vi "position sweep(SubVI).vi"(0 "data":refnum<queue>, 2 "Instrument Ref In":refnum<k24>, 4 "config":refnum<queue>, 5 "steps number":i32, 7 "ch str":string, 9 "Position":dbl=300.0, 12 "Resource In":refnum<visa-resource-name>, 13 "Position 2":dbl=300.0, 14 "Speed":i32=10 min=0 max=14) -> (8 "错误输出":errorcluster)   [LabVIEW 2019, in "SubVI.lvlib"]
uses:
  SubVI.lvlib
  lib/QDInstrument.dll
  config.ctl
panel:
  # "(真是通道1，假是通道2)"
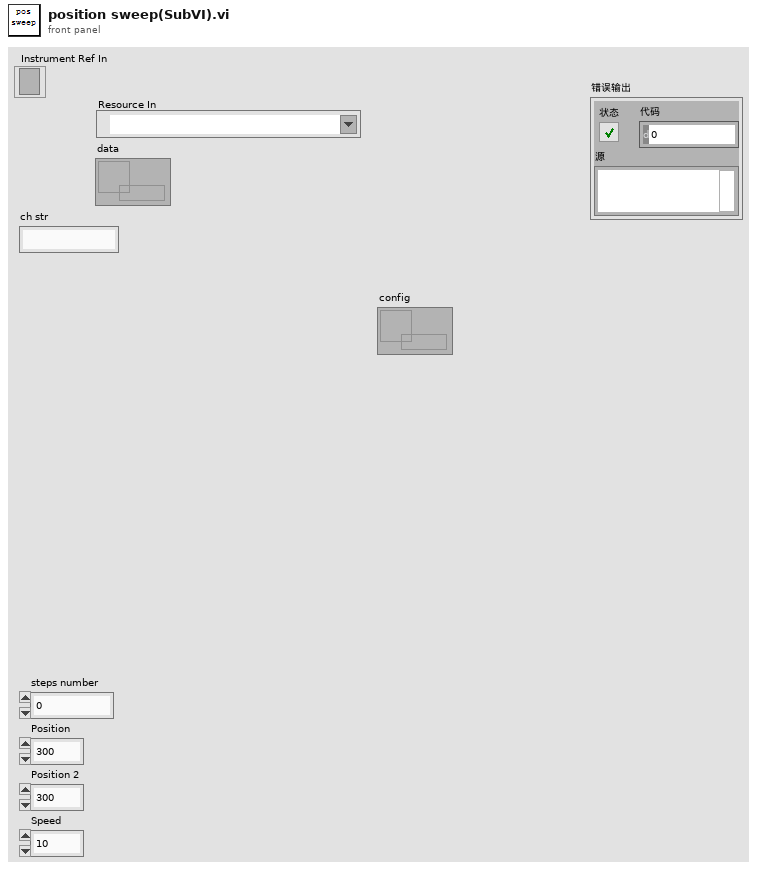
[diagram p1: front panel]
types:
  T1 = typedef "config.ctl" = cluster{"error":bool, "initialize":string, "数值":dbl, "6221":cluster{"6221 Resource":refnum<visa-resource-name>, "Delta status":bool}, "7001":cluster{"Ch":bool}}
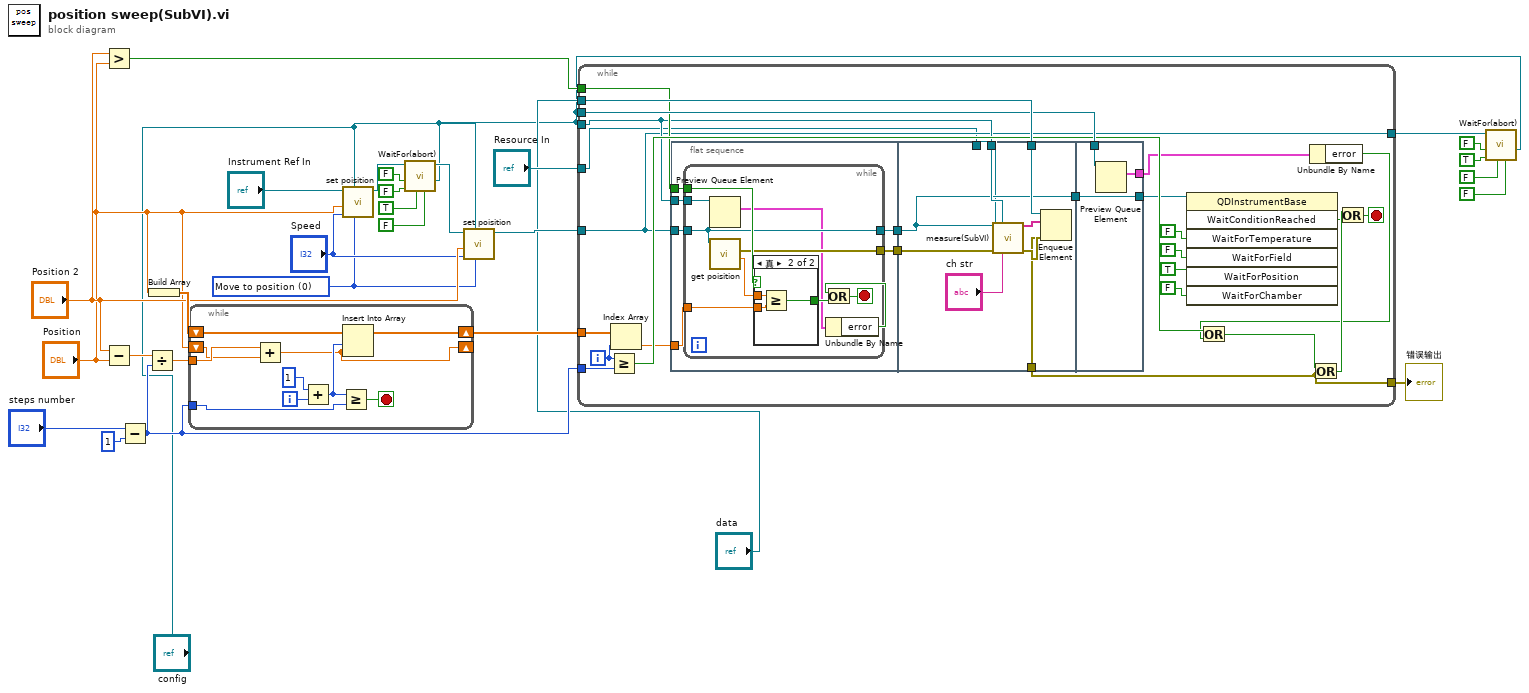
[diagram p0: block diagram]
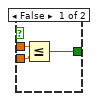
[diagram p2: hidden frame]
diagram:
  w4 = u16 0 items=["Move to position", "Move to limit", "Redefine current position"] ("Mode")
  n1 = Greater?(x="Position 2", y="Position") -> (0:w17:bool)
  n2 = Subtract(x="Position 2", y="Position") -> (x-y=w29:dbl)
  n3 = Subtract(x="steps number", y=1) -> (x-y=w6:i32)
  n4 = Divide(x=w29, y=w6) -> (x/y=w27:dbl)
  n5 = Build Array("Position") -> (w28:dbl[])
  n6 = while {
    shift-right: [w39] -> w19
    shift-left: w28 -> [w38]
    tunnel: w27 -> [w33]
    tunnel: w6 -> [w32]
    shift-right: [w31] -> _
    shift-left: "Position" -> [w30]
    i -> [w37]
    stop <- w34 stop-if-true
    n7 = Add(x=w33, y=w30) -> (x+y=w31:dbl)
    n8 = Add(x=1, y=w37) -> (x+y=w35:i32)
    n9 = Greater Or Equal?(x=w35, y=w32) -> (x >= y?=w34:bool)
    n10 = Insert Into Array(array=w38, index=w35, new element=w31) -> (w39:dbl[])
  }
  n11 = call "set poisition.vi"("Mode"=w4, "config"="config", "Slow down code\ndefault = 0"="Speed", "Position (deg)"="Position", "Instrument Ref In"="Instrument Ref In") -> ("Instrument Ref Out"=w5:refnum<k24>)  [unwired: 3 in, 1 out]
  n12 = call "WaitFor(abort).vi"("config"="config", "Wait For Chamber"=FALSE, "Wait For Position"=TRUE, "Wait For Field"=FALSE, "Wait For Temperature"=FALSE, "Instrument Ref In"=w5) -> ("Instrument Ref Out"=w20:refnum<k24>)  [unwired: 4 in, 1 out]
  n13 = call "set poisition.vi"("Mode"=w4, "config"="config", "Slow down code\ndefault = 0"="Speed", "Position (deg)"="Position 2", "Instrument Ref In"=w20) -> ("Instrument Ref Out"=w15:refnum<k24>)  [unwired: 3 in, 1 out]
  n14 = while {
    tunnel: w19 -> [w65]
    tunnel: w6 -> [w60]
    tunnel: "data" -> [w63]
    tunnel: "config" -> [w62]
    tunnel: w15 -> [w53]
    tunnel: w17 -> [w58]
    tunnel: [w53] -> w10
    tunnel: "config" -> [w56]
    tunnel: [w42] -> w9
    tunnel: "Resource In" -> [w43]
    i -> [w59]
    stop <- w47 stop-if-true
    n15 = Greater Or Equal?(x=w59, y=w60) -> (x >= y?=w61:bool)
    n16 = Index Array(array=w65, index=w59) -> (element=w57:dbl)
    n17 = flat-sequence {
      tunnel: [w68] -> w64
      tunnel: w53 -> [w71]
      tunnel: w58 -> [w70]
      tunnel: w57 -> [w69]
      tunnel: w56 -> [w67]
      tunnel: [w66] -> w55
      tunnel: w64 -> [w93]
      tunnel: w63 -> [w96]
      tunnel: w56 -> [w95]
      tunnel: [w89] -> w42
      tunnel: w55 -> [w91]
      tunnel: [w93] -> w51
      tunnel: w43 -> [w92]
      tunnel: w62 -> [w99]
      tunnel: [w98] -> w41
      tunnel: [w97] -> w52
      tunnel: w51 -> [w97]
      frame #0 {
        n18 = while {
          tunnel: w71 -> [w79]
          tunnel: w70 -> [w81]
          tunnel: w69 -> [w80]
          tunnel: [w79] -> w68
          tunnel: w67 -> [w77]
          tunnel: [w75] -> w66
          stop <- w72 stop-if-true
          n19 = Preview Queue Element(queue=w77) -> (element=w74:T1)  [unwired: 2 in, 3 out]
          n20 = call "get poisition.vi"("Instrument Ref In"=w79) -> ("Position"=w78:dbl, "error out"=w75:errorcluster)  [unwired: 4 in, 1 out]
          n21 = case shown="真" w81 {
            tunnel: w78 -> [w84 w87]
            tunnel: w80 -> [w83 w86]
            tunnel: [w82 w85] -> w76
            frame False {
              n22 = Less Or Equal?(x=w84, y=w83) -> (x <= y?=w82:bool)
            }
            frame True {
              n23 = Greater Or Equal?(x=w87, y=w86) -> (x >= y?=w85:bool)
            }
          }
          n24 = Unbundle By Name(w74) -> ("error"=w73:bool)
          n25 = Or(x=w73, y=w76) -> (x .or. y?=w72:bool)
        }
      }
      frame #1 {
        n26 = call "measure(SubVI).vi"(".NET引用句柄输入"=w93, "config"=w95, 7:w92, "error in (no error)"=w91, "ch str"="ch str") -> ("data"=w94:string[], "error out"=w90:errorcluster)  [unwired: 9 in]
        n27 = Enqueue Element(queue=w96, element=w94, error in (no error)=w90) -> (error out=w89:errorcluster)  [unwired: 1 in, 2 out]
      }
      frame #2 {
        n28 = Preview Queue Element(queue=w99) -> (element=w98:T1)  [unwired: 2 in, 3 out]
      }
    }
    n29 = invoke class="QDInstrumentBase" method="WaitConditionReached"(reference=w52, "WaitForTemperature"=FALSE, "WaitForField"=FALSE, "WaitForPosition"=TRUE, "WaitForChamber"=FALSE) -> ("WaitConditionReached"=w48:bool)  [unwired: 2 in, 6 out]
    n30 = Unbundle By Name(w41) -> ("error"=w40:bool)
    n31 = Or(x=w61, y=w40) -> (x .or. y?=w54:bool)
    n32 = Or(x=w54, y=w42) -> (x .or. y?=w49:bool)
    n33 = Or(x=w49, y=w48) -> (x .or. y?=w47:bool)
  }
  "错误输出" <- w9
  n34 = call "WaitFor(abort).vi"("config"="config", "Wait For Chamber"=FALSE, "Wait For Position"=FALSE, "Wait For Field"=TRUE, "Wait For Temperature"=FALSE, "Instrument Ref In"=w10) -> ()  [unwired: 4 in, 2 out]
